vi "ResponseTimeTest.vi"() -> ()   [LabVIEW 2018, in "AltonTech MALT200817.lvlib"]
uses:
  AltonTech MALT200817.lvlib
panel:
  out "Write Read Time (ms)":u32
  out "Total Time":u32
  out "data out":string
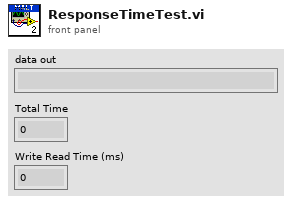
[diagram p1: front panel]
types:
  T1 = enum16{"Standard", "Buffered", "CRLF", "Immediate"}
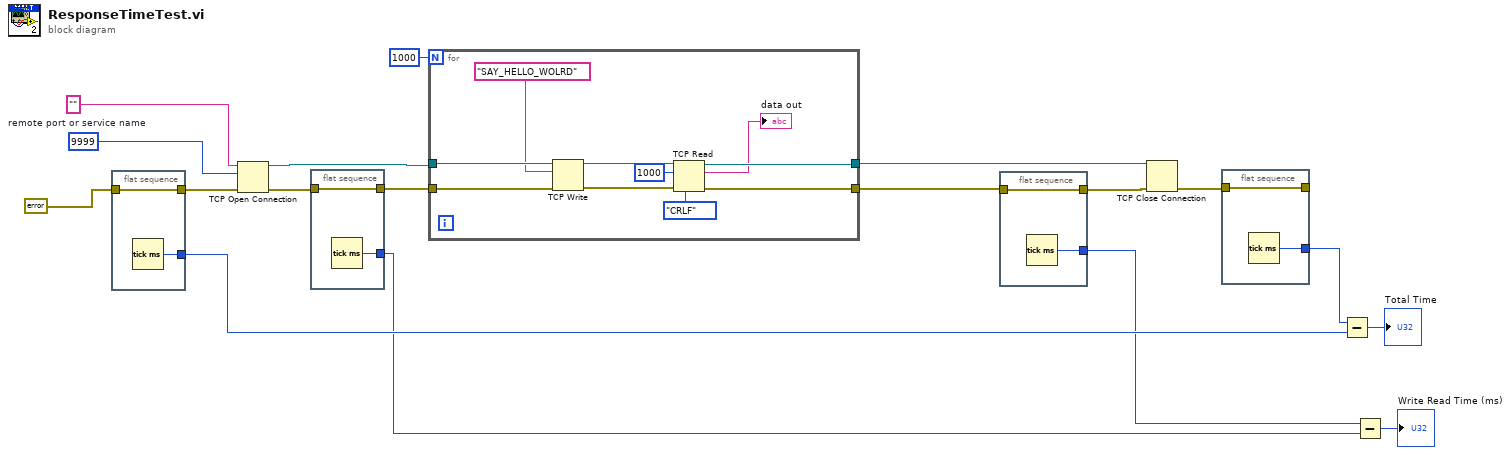
[diagram p0: block diagram]
diagram:
  w13 = u16 9999  # remote port or service name
  n1 = flat-sequence {
    tunnel: errorcluster {"status"=FALSE, "code"=0, "source"=""} ("error in (no error)") -> [w20]
    tunnel: [w20] -> w14
    tunnel: [w19] -> w12
    frame #0 {
      n2 = Tick Count (ms)() -> (millisecond timer value=w19:u32)
    }
  }
  n3 = TCP Open Connection(address="", remote port or service name=w13, error in (no error)=w14) -> (connection ID=w18:refnum<k5>, error out=w10:errorcluster)  [unwired: 2 in]
  n4 = flat-sequence {
    tunnel: w10 -> [w22]
    tunnel: [w22] -> w9
    tunnel: [w21] -> w2
    frame #0 {
      n5 = Tick Count (ms)() -> (millisecond timer value=w21:u32)
    }
  }
  n6 = for {
    N: 1000 -> [_]
    tunnel: w18 -> [w32]
    tunnel: [w30] -> w17
    tunnel: w9 -> [w24]
    tunnel: [w23] -> w5
    n7 = TCP Write(connection ID=w32, data in="SAY_HELLO_WOLRD", error in (no error)=w24) -> (connection ID out=w31:refnum<k5>, error out=w25:errorcluster)  [unwired: 1 in, 1 out]
    n8 = TCP Read(connection ID=w31, bytes to read=1000, error in (no error)=w25, 7:T1."CRLF" ("mode (standard)")) -> (connection ID out=w30:refnum<k5>, data out=→"data out":string, error out=w23:errorcluster)  [unwired: 1 in]
  }
  n9 = flat-sequence {
    tunnel: w5 -> [w34]
    tunnel: [w34] -> w4
    tunnel: [w33] -> w3
    frame #0 {
      n10 = Tick Count (ms)() -> (millisecond timer value=w33:u32)
    }
  }
  n11 = TCP Close Connection(connection ID=w17, error in (no error)=w4) -> (error out=w8:errorcluster)  [unwired: 1 in, 1 out]
  n12 = flat-sequence {
    tunnel: w8 -> [w36]
    tunnel: [w36] -> _
    tunnel: [w35] -> w7
    frame #0 {
      n13 = Tick Count (ms)() -> (millisecond timer value=w35:u32)
    }
  }
  n14 = Subtract(x=w7, y=w12) -> (x-y=→"Total Time":u32)
  n15 = Subtract(x=w3, y=w2) -> (x-y=→"Write Read Time (ms)":u32)
